vi "Walk Up to File.vi"(8 "error in (no error)":errorcluster, 10 "name or relative path":string="file.txt", 11 "Start Path":path) -> (0 "error out":errorcluster, 2 "File Directory":path, 3 "File Path":path)   [LabVIEW 2019]
uses:
  <vilib>/Utility/error.llb/Error Cluster From Error Code.vi
  <vilib>/ErrorRing/Error Ring.xnode
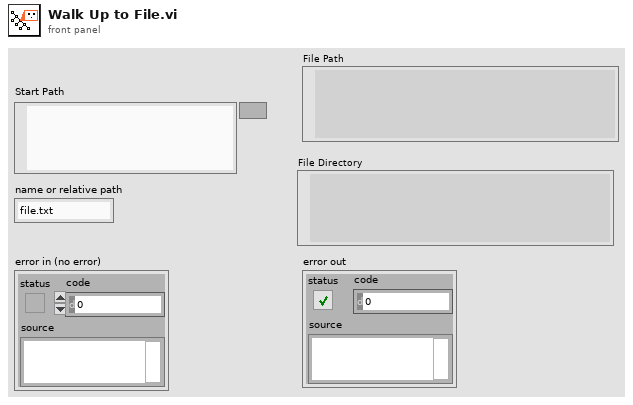
[diagram p1: front panel]
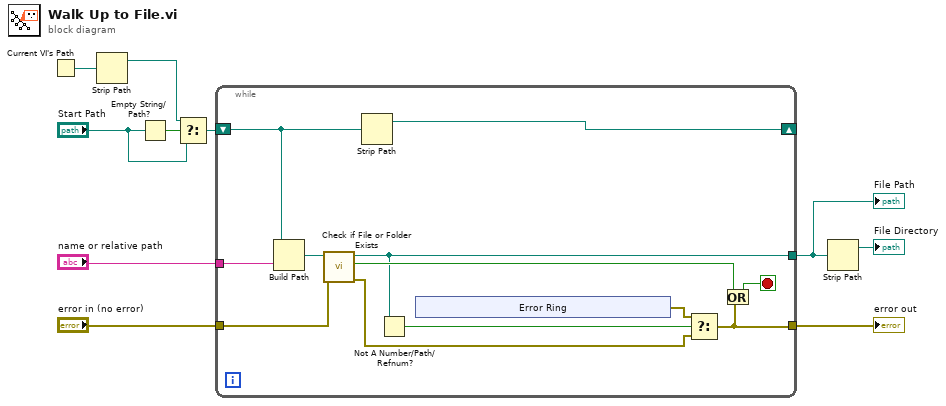
[diagram p0: block diagram]
diagram:
  n1 = Current VI's Path() -> (path=w6:path)
  n2 = Strip Path(path=w6) -> (stripped path=w2:path)  [unwired: 1 out]
  n3 = Empty String/Path?(string/path="Start Path") -> (empty?=w3:bool)
  n4 = Select(t=w2, s=w3, f="Start Path") -> (s? t:f=w4:path)
  n5 = while {
    shift-right: [w22] -> _
    shift-left: w4 -> [w21]
    tunnel: [w13] -> w5
    tunnel: "error in (no error)" -> [w12]
    tunnel: [w14] -> w9
    tunnel: "name or relative path" -> [w11]
    stop <- w17 stop-if-true
    n6 = Build Path(base path=w21, name or relative path=w11) -> (appended path=w20:path)
    n7 = call <vilib>:"Check if File or Folder Exists.vi"("error in (no error)"=w12, "path"=w20) -> ("error out"=w15:errorcluster, "file or folder exists?"=w18:bool, "dup path"=w13:path)  [unwired: 7 in]
    n8 = Strip Path(path=w21) -> (stripped path=w22:path)  [unwired: 1 out]
    n9 = Not A Number/Path/Refnum?(number/path/refnum=w13) -> (NaN/Path/Refnum?=w19:bool)
    n10 = xnode "Error Ring"() -> ("error out"=w16:errorcluster)
    n11 = Select(t=w16, s=w19, f=w15) -> (s? t:f=w14:errorcluster)
    n12 = Or(x=w18, y=w14) -> (x .or. y?=w17:bool)
  }
  "error out" <- w9
  "File Path" <- w5
  n13 = Strip Path(path=w5) -> (stripped path=→"File Directory":path)  [unwired: 1 out]
